vi "_Debug+344.vi"() -> ()   [LabVIEW 2017]
uses:
  <vilib>/Instr/_visa.llb/VISA Configure Serial Port (Instr).vi
  <instrlib>/Agilent 34401/Public/Data/Read (Single Point).vi
  <instrlib>/Agilent 34401/Agilent 34401.lvlib
panel:
  out "Vdac/Vch1":cluster{dbl[], dbl[]}(graph)
  out "Numeric":i32
  out "Vdac/Vout":cluster{dbl[], dbl[]}(graph)
  out "344":cluster{dbl[], dbl[]}(graph)
  out "DAC1":cluster{dbl[], dbl[]}(graph)
  out "Current344, mA":dbl format="%#_4g"
  in  "COM 344":refnum<visa-resource-name>
  out "DAC1volt, V":dbl
  out "Bytes at Port":u32
  out "RecTry":i32
  out "OutVoltage, V":dbl
  out "Knob":u32
  out "Current, mA":dbl format="%#_4g"
  out "Channel 1, V":dbl format="%#_5g"
  in  "Stop Button":bool
  in  "Start Button":bool
  out "VoltageArray, V":dbl[](array[numeric])
  in  "Step, V":dbl
  in  "Amplitude, V":dbl
  in  "LOG file":path
  in  "COM port":refnum<visa-resource-name>
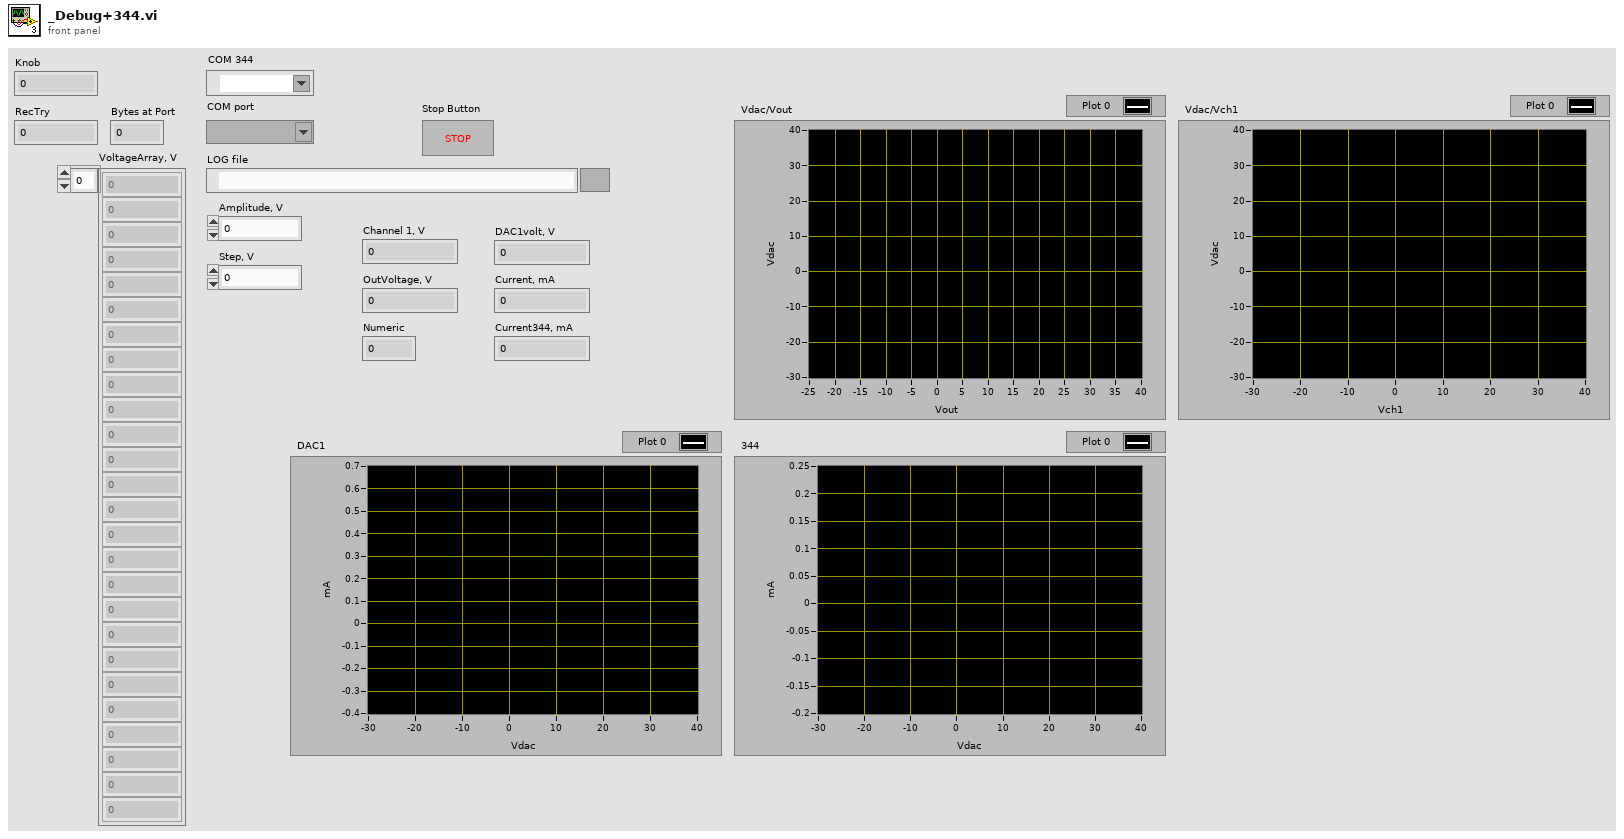
[diagram p1: front panel]
types:
  T1 = cluster{"Baud Rate":u32, "Parity":u16, "Data Bits":u16}
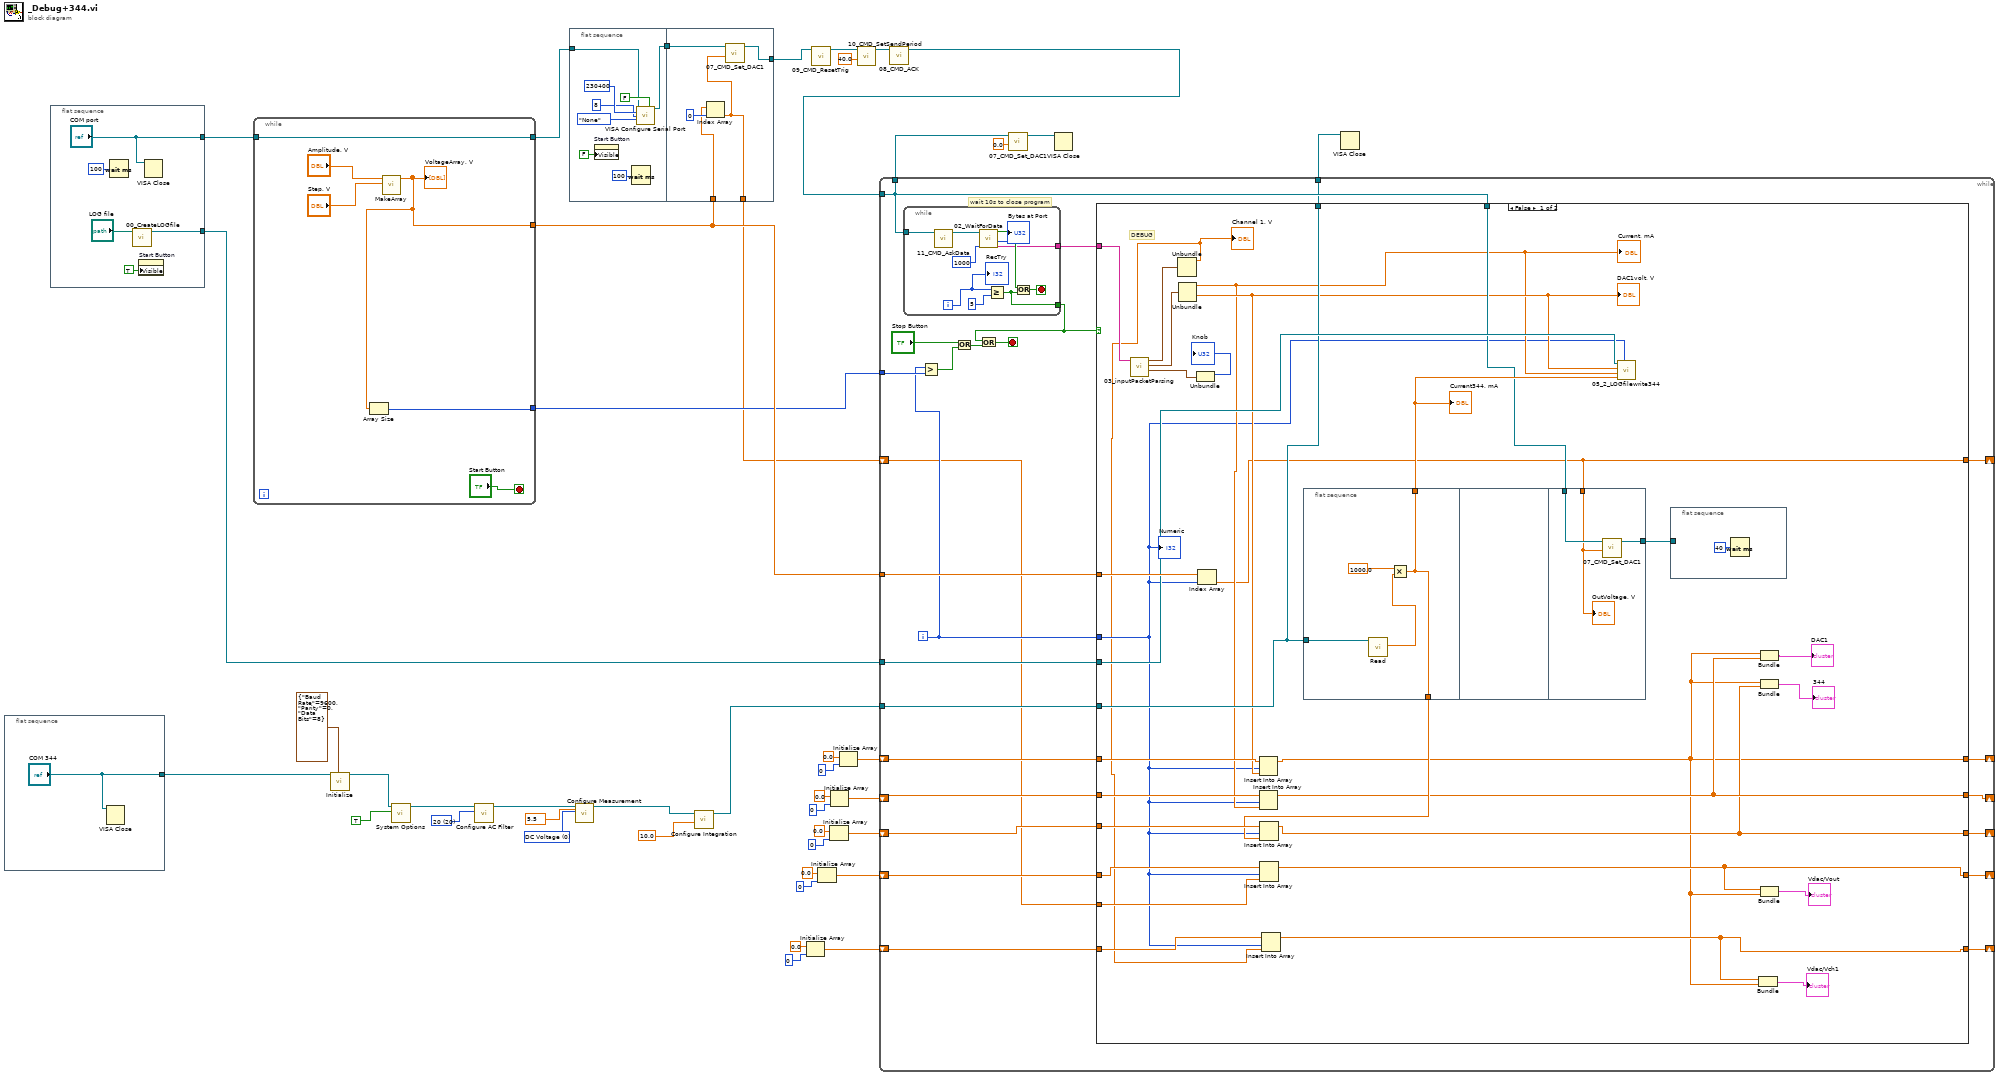
[diagram p0: block diagram]
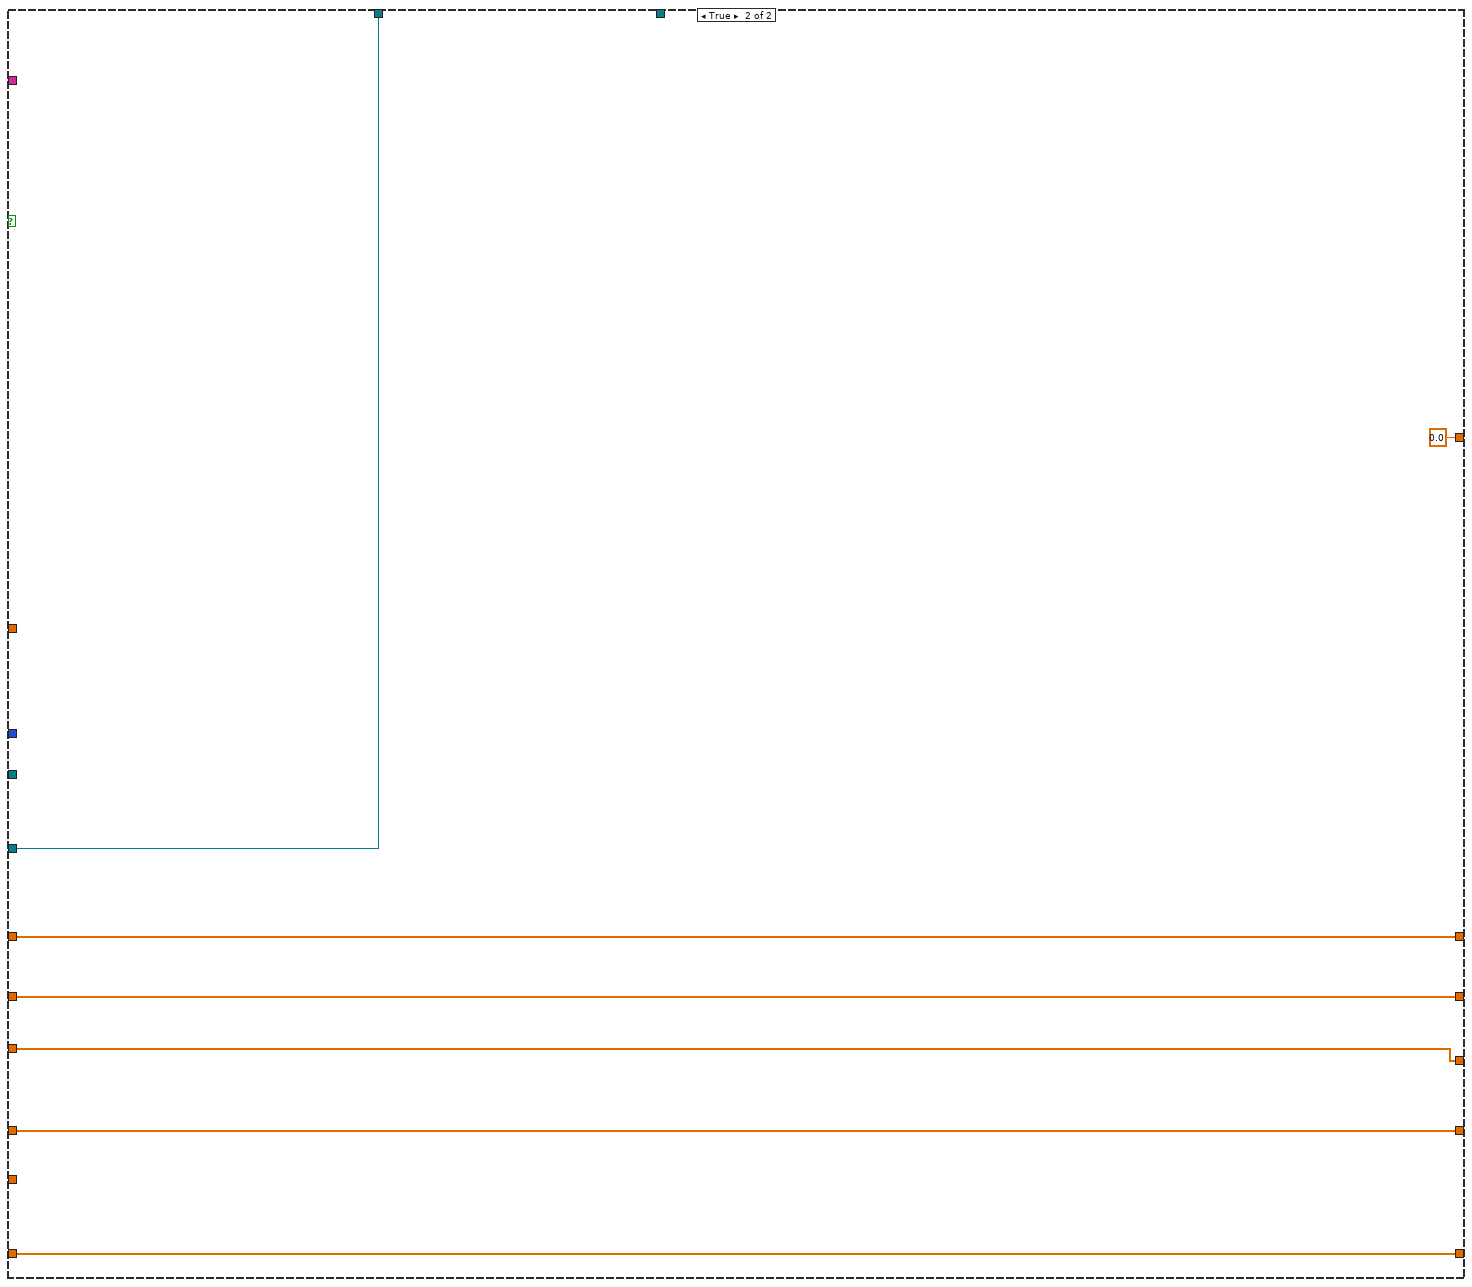
[diagram p2: hidden frame]
diagram:
  w20 = 10.0 items=["0.001"=0.001, "0.002"=0.002, "0.006"=0.006, "0.02"=0.02, "0.06"=0.06, "0.2"=0.2, "1"=1.0, "10"=10.0, "100"=100.0] ("Integration Time (1 PLCs)")
  w26 = 20 items=["3"=3, "20"=20, "200"=200] ("AC Filter Bandwidth (20 Hz)")
  w27 = u16 0 items=["DC Voltage", "AC Voltage", "2 - Wire Resistance", "4 - Wire Resistance", "DC Current", "AC Current", "Frequency", "Period", "Continuity", "Diode Checking", "VDC:VDC Ratio", "Temperature", "Capacitance"] ("Function (0: DC Voltage)")
  w28 = 5.5 items=["4.5"=4.5, "5.5"=5.5, "6.5"=6.5] ("Manual Resolution (5.5 Digits)")
  n1 = flat-sequence {
    tunnel: ["COM 344"] -> w21
    frame #0 {
      n2 = VISA Close(VISA resource name="COM 344") -> ()  [unwired: 1 in, 1 out]
    }
  }
  n3 = flat-sequence {
    tunnel: ["COM port"] -> w43
    tunnel: [w46] -> w41
    frame #0 {
      n4 = Wait (ms)(milliseconds to wait=u32 100) -> ()  [unwired: 1 out]
      n5 = call "00_CreateLOGfile.vi"("LOG file"="LOG file") -> ("refnum out"=w46:refnum<file>)  [unwired: 10 in]
      n6 = property on="Start Button" class="Bool"("Visible"=TRUE) -> ()  [unwired: 2 in, 2 out]
      n7 = VISA Close(VISA resource name="COM port") -> ()  [unwired: 1 in, 1 out]
    }
  }
  n8 = while {
    tunnel: w43 -> [w52]
    tunnel: [w52] -> w42
    tunnel: [w51] -> w31
    tunnel: [w50] -> w30
    stop <- "Start Button" stop-if-true
    n9 = call "MakeArray.vi"("Amp"="Amplitude, V", "Step"="Step, V") -> ("Array"=w51:dbl[])  [unwired: 8 in]
    "VoltageArray, V" <- w51
    n10 = Array Size(array=w51) -> (size(s)=w50:i32)
  }
  n11 = call <instrlib>:"Initialize.vi"("Serial Configuration"=T1 {"Baud Rate"=9600, "Parity"=0, "Data Bits"=8}, "VISA resource name"=w21) -> ("VISA resource name out"=w23:refnum<visa-resource-name>)  [unwired: 8 in, 1 out]
  n12 = call <instrlib>:"System Options.vi"("Display (T: On)"=TRUE, "VISA resource name"=w23) -> ("VISA resource name out"=w24:refnum<visa-resource-name>)  [unwired: 8 in, 1 out]
  n13 = call <instrlib>:"Configure AC Filter.vi"("AC Filter Bandwidth (20 Hz)"=w26, "VISA resource name"=w24) -> ("VISA resource name out"=w25:refnum<visa-resource-name>)  [unwired: 8 in, 1 out]
  n14 = flat-sequence {
    tunnel: w42 -> [w59]
    tunnel: [w58] -> w32
    tunnel: [w67] -> w39
    tunnel: w32 -> [w66]
    tunnel: w31 -> [w65]
    tunnel: [w64] -> w4
    frame #0 {
      n15 = property on="Start Button" class="Bool"("Visible"=FALSE) -> ()  [unwired: 2 in, 2 out]
      n16 = Wait (ms)(milliseconds to wait=u32 100) -> ()  [unwired: 1 out]
      n17 = call-poly "VISA Configure Serial Port"("VISA resource name"=w59, "Enable Termination\nChar (T)"=FALSE ("Enable Termination\nChar (T)"), "baud rate (9600)"=u32 230400, "data bits (8)"=u16 8, "parity (0:none)"=enum16{"None", "Odd", "Even", "Mark", "Space"}."None") -> ("VISA resource name out"=w58:refnum<visa-resource-name>)  [unwired: 9 in, 1 out]
    }
    frame #1 {
      n18 = Index Array(array=w65, index=0) -> (element=w64:dbl)
      n19 = call "07_CMD_Set_DAC1.vi"("Input, V"=w64, "VISA resource name"=w66) -> ("VISA resource name out"=w67:refnum<visa-resource-name>)  [unwired: 9 in]
    }
  }
  n20 = call <instrlib>:"Configure Measurement.vi"("Manual Resolution (5.5 Digits)"=w28, "Function (0: DC Voltage)"=w27, "VISA resource name"=w25) -> ("VISA resource name out"=w19:refnum<visa-resource-name>)  [unwired: 7 in, 1 out]
  n21 = call <instrlib>:"Configure Integration.vi"("Integration Time (1 PLCs)"=w20, "VISA resource name"=w19) -> ("VISA resource name out"=w18:refnum<visa-resource-name>)  [unwired: 8 in, 1 out]
  n22 = Initialize Array(0.0 ("element"), 0 ("dimension size")) -> (w1:dbl[])
  n23 = call "09_CMD_ResetTrig.vi"("VISA resource name"=w39) -> ("VISA resource name out"=w35:refnum<visa-resource-name>)  [unwired: 10 in]
  n24 = Initialize Array(0.0 ("element"), 0 ("dimension size")) -> (w5:dbl[])
  n25 = Initialize Array(0.0 ("element"), 0 ("dimension size")) -> (w8:dbl[])
  n26 = Initialize Array(0.0 ("element"), 0 ("dimension size")) -> (w11:dbl[])
  n27 = Initialize Array(0.0 ("element"), 0 ("dimension size")) -> (w16:dbl[])
  n28 = call "10_CMD_SetSendPeriod.vi"("Period, ms"=40.0, "VISA resource name"=w35) -> ("VISA resource name out"=w34:refnum<visa-resource-name>)  [unwired: 9 in]
  n29 = call "08_CMD_ACK.vi"("VISA resource name"=w34) -> ("VISA resource name out"=w33:refnum<visa-resource-name>)  [unwired: 10 in]
  n30 = while {
    tunnel: w33 -> [w88]
    tunnel: [w88] -> w40
    tunnel: w31 -> [w89]
    tunnel: w41 -> [w90]
    tunnel: w30 -> [w85]
    tunnel: w18 -> [w82]
    tunnel: [w81] -> w17
    shift-right: [w77] -> _
    shift-left: w16 -> [w78]
    shift-right: [w76] -> _
    shift-left: w11 -> [w79]
    shift-right: [w75] -> _
    shift-left: w8 -> [w80]
    shift-right: [w73] -> _
    shift-left: w5 -> [w74]
    shift-right: [w72] -> _
    shift-left: w4 -> [w71]
    shift-right: [w69] -> _
    shift-left: w1 -> [w70]
    i -> [w83]
    stop <- w93 stop-if-true
    # "wait 10s to close program"
    n31 = while {
      tunnel: w88 -> [w141]
      tunnel: [w145] -> w92
      tunnel: [w146] -> w91
      i -> [w144]
      stop <- w148 stop-if-true
      n32 = call "11_CMD_AskData.vi"("VISA resource name"=w141) -> ("VISA resource name out"=w142:refnum<visa-resource-name>)  [unwired: 10 in]
      n33 = call "02_WaitForData.vi"("WaitTimeoutMS"=u32 1000, "VISA"=w142) -> ("Buffer"=w146:string, "Bytes at Port"=→"Bytes at Port":u32, "Data Recived"=w147:bool)  [unwired: 7 in]
      n34 = Greater Or Equal?(x=w144, y=5) -> (x >= y?=w145:bool)
      n35 = Or(x=w147, y=w145) -> (x .or. y?=w148:bool)
      "RecTry" <- w144
    }
    n36 = Greater?(x=w83, y=w85) -> (0:w84:bool)
    n37 = Or(x="Stop Button", y=w84) -> (x .or. y?=w87:bool)
    n38 = Or(x=w92, y=w87) -> (x .or. y?=w93:bool)
    n39 = case shown="False" w92 {
      tunnel: w91 -> [w118 _]
      tunnel: w90 -> [w119 _]
      tunnel: w83 -> [w99 _]
      tunnel: w89 -> [w121 _]
      tunnel: w88 -> [w117 _]
      tunnel: w82 -> [w116 w140]
      tunnel: [w116 w140] -> w81
      tunnel: w80 -> [w115 w137]
      tunnel: w79 -> [w114 w138]
      tunnel: w78 -> [w113 w139]
      tunnel: [w94 w139] -> w77
      tunnel: [w109 w138] -> w76
      tunnel: [w108 w137] -> w75
      tunnel: w74 -> [w105 w136]
      tunnel: [w96 w136] -> w73
      tunnel: [w104 0.0] -> w72
      tunnel: w71 -> [w103 _]
      tunnel: w70 -> [w100 w134]
      tunnel: [w95 w134] -> w69
      frame False {
        # "DEBUG"
        n40 = call "03_inputPacketParsing.vi"("string"=w118) -> ("Service state"=w122:cluster{u8, u8}, "DAC state"=w125:cluster{dbl, dbl, dbl, dbl}, "Voltage"=w123:cluster{dbl, dbl, dbl, dbl})  [unwired: 7 in, 1 out]
        n41 = Unbundle(w123) -> (w98:dbl)  [unwired: 3 out]
        "Channel 1, V" <- w98
        n42 = Unbundle(w125) -> (w111:dbl, w112:dbl)  [unwired: 2 out]
        "Current, mA" <- w111
        "DAC1volt, V" <- w112
        n43 = Unbundle(w122) -> (→"Knob":u8)  [unwired: 1 out]
        n44 = Index Array(array=w121, index=w99) -> (element=w104:dbl)
        n45 = Insert Into Array(array=w113, index=w99, new element=w112) -> (w94:dbl[])
        n46 = Insert Into Array(array=w114, index=w99, new element=w111) -> (w109:dbl[])
        n47 = Insert Into Array(array=w115, index=w99, new element=w110) -> (w108:dbl[])
        n48 = Insert Into Array(array=w105, index=w99, new element=w103) -> (w96:dbl[])
        n49 = Insert Into Array(array=w100, index=w99, new element=w98) -> (w95:dbl[])
        n50 = flat-sequence {
          tunnel: w116 -> [w130]
          tunnel: [w127] -> w120
          tunnel: [w127] -> w110
          tunnel: w104 -> [w131]
          tunnel: w117 -> [w133]
          tunnel: [w132] -> w101
          frame #0 {
            n51 = call-poly <instrlib>:"Read.vi"("VISA resource name"=w130) -> ("Measurement"=w129:dbl)  [unwired: 8 in, 2 out]
            n52 = Multiply(x=1000.0, y=w129) -> (x*y=w127:dbl)
          }
          frame #1 {
          }
          frame #2 {
            n53 = call "07_CMD_Set_DAC1.vi"("Input, V"=w131, "VISA resource name"=w133) -> ("VISA resource name out"=w132:refnum<visa-resource-name>)  [unwired: 9 in]
            "OutVoltage, V" <- w131
          }
        }
        n54 = call "05_2_LOGfilewrite344.vi"("N"=w99, "344cur"=w120, "DAC1cur"=w111, "DAC1volt2"=w112, "refnum out"=w119) -> ()  [unwired: 7 in]
        n55 = flat-sequence {
          tunnel: w101 -> [_]
          frame #0 {
            n56 = Wait (ms)(milliseconds to wait=u32 40) -> ()  [unwired: 1 out]
          }
        }
        n57 = Bundle(w95, w94) -> (→"Vdac/Vch1":cluster{dbl[], dbl[]})  [unwired: 1 in]
        n58 = Bundle(w94, w109) -> (→"DAC1":cluster{dbl[], dbl[]})  [unwired: 1 in]
        n59 = Bundle(w94, w108) -> (→"344":cluster{dbl[], dbl[]})  [unwired: 1 in]
        n60 = Bundle(w96, w94) -> (→"Vdac/Vout":cluster{dbl[], dbl[]})  [unwired: 1 in]
        "Current344, mA" <- w120
        "Numeric" <- w99
      }
      frame True {
      }
    }
  }
  n61 = call "07_CMD_Set_DAC1.vi"("Input, V"=0.0, "VISA resource name"=w40) -> ("VISA resource name out"=w37:refnum<visa-resource-name>)  [unwired: 9 in]
  n62 = VISA Close(VISA resource name=w37) -> ()  [unwired: 1 in, 1 out]
  n63 = VISA Close(VISA resource name=w17) -> ()  [unwired: 1 in, 1 out]
